vi "Set KH Cluster From UI Array.vi"(8 "error in (no error)":errorcluster, 9 "Number of AI":i32=1, 10 "UI Channels []":T9[](array[typedef]) {"KH"."Channel" items=["A 1"]}, 11 "KH Cluster":T1) -> (0 "error out":errorcluster, 3 "KH Cluster out":T1)   [LabVIEW 2019, in "SMO.Control Experiment UI.lvclass"]
uses:
  SMO.Control Experiment UI.lvclass
  Typedefs/UI Channels--Cluster.ctl
  Typedefs/UI Channels.AI--Cluster.ctl
  Typedefs/UI Channels.Device--Cluster.ctl
  Control Experiment/Typedefs/KH Mode-enum.ctl
  Typedefs/UI Channels.KH--Cluster.ctl
  <userlib>/LevyLab/Krohn Hite 7008/typedefs/Input Configuration-Enum.ctl
  <userlib>/LevyLab/Krohn Hite 7008/typedefs/Gain-Enum.ctl
  <userlib>/LevyLab/Krohn Hite 7008/typedefs/Shunt-Enum.ctl
  Typedefs/UI Channels.AO--Cluster.ctl
  Typedefs/KH Cluster--Cluster.ctl
  <userlib>/LevyLab/Krohn Hite 7008/typedefs/SetAll-Cluster.ctl
  <userlib>/LevyLab/Krohn Hite 7008/typedefs/Channel-Enum.ctl
  <userlib>/LevyLab/Krohn Hite 7008/typedefs/Filter-Enum.ctl
  <userlib>/LevyLab/Krohn Hite 7008/typedefs/Coupling-Enum.ctl
  Control Experiment/Control Experiment.lvclass
  <userlib>/LevyLab/Krohn Hite 7008/Instrument.KH7008.lvclass
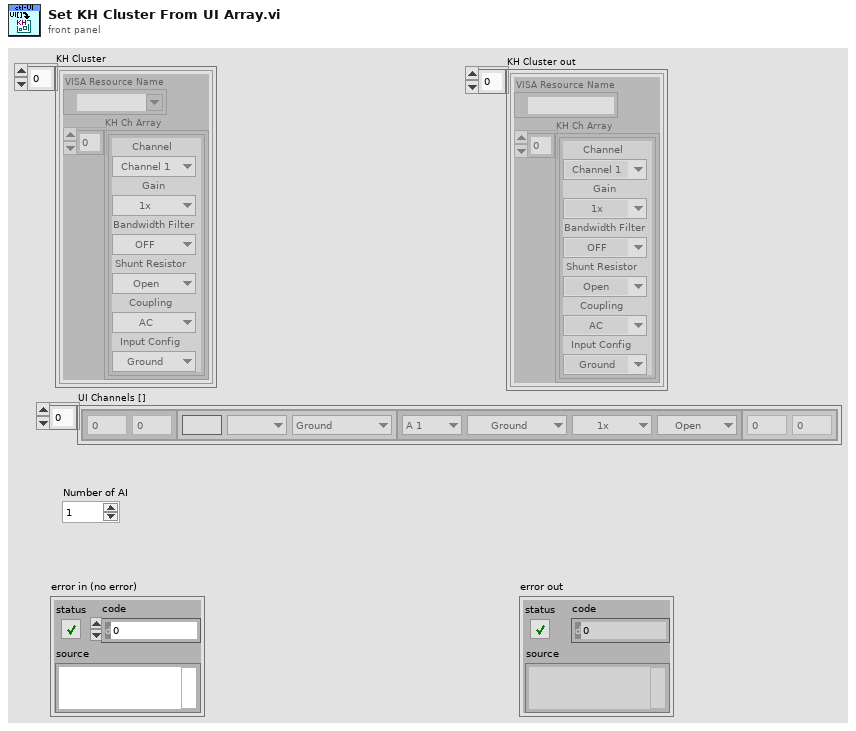
[diagram p1: front panel]
types:
  T1 = typedef "SMO.Control Experiment UI.lvclass/KH Cluster--Cluster.ctl" = cluster{"VISA Resource Name":refnum<visa-resource-name>, "KH Ch Array":T2[]}[]
  T2 = typedef "Instrument.KH7008.lvclass/SetAll-Cluster.ctl" = cluster{"Channel":T3, "Gain":T4, "Bandwidth Filter":T5, "Shunt Resistor":T6, "Coupling":T7, "Input Config":T8}
  T3 = typedef "Instrument.KH7008.lvclass/Channel-Enum.ctl" = enum16{"Channel 1", "Channel 2", "Channel 3", "Channel 4", "Channel 5", "Channel 6", "Channel 7", "Channel 8"}
  T4 = typedef "Instrument.KH7008.lvclass/Gain-Enum.ctl" = enum16{"1x", "10x", "100x", "1000x"}
  T5 = typedef "Instrument.KH7008.lvclass/Filter-Enum.ctl" = enum16{"OFF", "ON"}
  T6 = typedef "Instrument.KH7008.lvclass/Shunt-Enum.ctl" = enum16{"Open", "50 Ohms", "500 Ohms", "5k Ohms", "50k Ohms", "10M Ohm"}
  T7 = typedef "Instrument.KH7008.lvclass/Coupling-Enum.ctl" = enum16{"AC", "DC"}
  T8 = typedef "Instrument.KH7008.lvclass/Input Configuration-Enum.ctl" = enum16{"Ground", "SE+ (-gnd)", "SE- (+gnd)", "Differential"}
  T9 = typedef "SMO.Control Experiment UI.lvclass/UI Channels--Cluster.ctl" = cluster{"AI":T10, "Device":T11, "KH":T13, "AO":T14}
  T10 = typedef "SMO.Control Experiment UI.lvclass/UI Channels.AI--Cluster.ctl" = cluster{"Channel":u32, "Gain":dbl}
  T11 = typedef "SMO.Control Experiment UI.lvclass/UI Channels.Device--Cluster.ctl" = cluster{"Electrode":string, "Configuration":T12, "Label":u16}
  T12 = typedef "Control Experiment.lvclass/KH Mode-enum.ctl" = enum16{"Ground", "Current", "Voltage (SE)", "Voltage (Diff)", "Gate"}
  T13 = typedef "SMO.Control Experiment UI.lvclass/UI Channels.KH--Cluster.ctl" = cluster{"Channel":u16, "Configuration":T8, "Gain":T4, "Shunt Resistor":T6}
  T14 = typedef "SMO.Control Experiment UI.lvclass/UI Channels.AO--Cluster.ctl" = cluster{"Channel":u32, "Gain":dbl}
  T15 = cluster{"VISA Resource Name":refnum<visa-resource-name>, "KH Ch Array":T2[]}
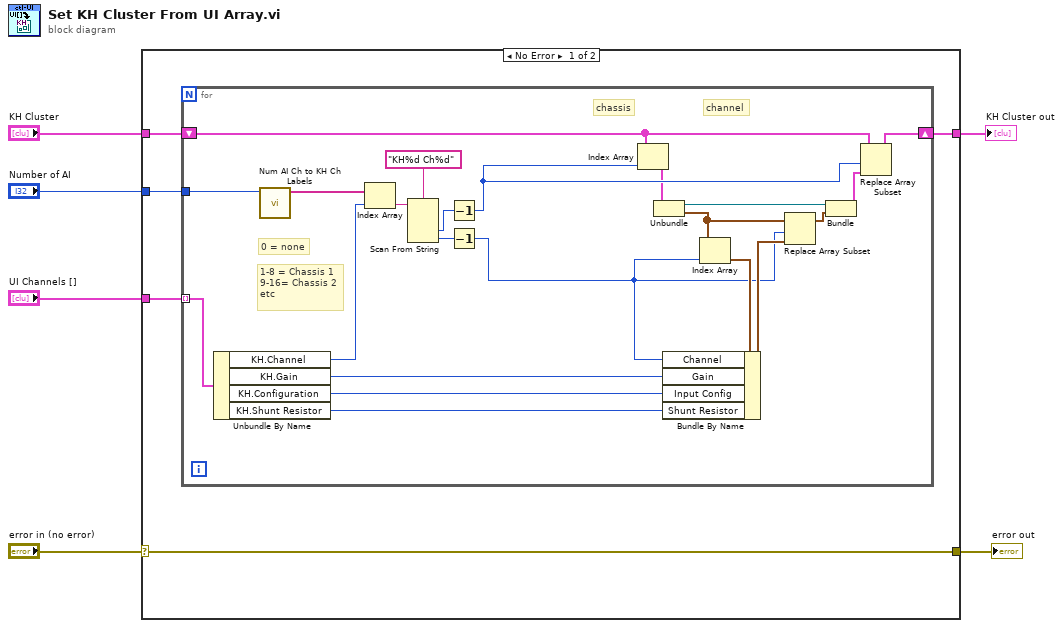
[diagram p0: block diagram]
diagram:
  n1 = case shown="No Error" "error in (no error)" {
    selector: "error in (no error)" -> [w7 w35]
    tunnel: [w11 w34] -> w6
    tunnel: "UI Channels []" -> [w10 _]
    tunnel: "Number of AI" -> [w9 _]
    tunnel: "KH Cluster" -> [w8 w34]
    tunnel: [w7 w35] -> w1
    frame No Error {
      n2 = for {
        tunnel: w10 -> [w20] mode=indexing
        shift-right: [w33] -> w11
        shift-left: w8 -> [w32]
        tunnel: w9 -> [w17]
        # "1-8 = Chassis 1\n9-16= Chassis 2\netc"
        # "0 = none"
        # "channel"
        # "chassis"
        n3 = Unbundle By Name(w20) -> ("KH.Channel"=w19:u16, "KH.Gain"=w21:T4, "KH.Configuration"=w22:T8, "KH.Shunt Resistor"=w23:T6)
        n4 = call "Num AI Ch to KH Ch Labels.vi"("Number of AI"=w17) -> ("KH Ch []"=w18:string[])  [unwired: 9 in, 1 out]
        n5 = Index Array(array=w18, index=w19) -> (element=w29:string)
        n6 = Scan From String(format string="KH%d Ch%d", input string=w29) -> (output 1=w28:i32, output 2=w27:i32)  [unwired: 4 in, 3 out]
        n7 = Decrement(x=w28) -> (x-1=w25:i32)
        n8 = Decrement(x=w27) -> (x-1=w24:i32)
        n9 = Index Array(array=w32, index=w25) -> (element=w15:T15)
        n10 = Unbundle(w15) -> ("VISA Resource Name"=w13:refnum<visa-resource-name>, "KH Ch Array"=w16:T2[])
        n11 = Index Array(array=w16, index=w24) -> (element=w31:T2)
        n12 = Bundle By Name(cluster=w31, "Channel"=w24, "Gain"=w21, "Input Config"=w22, "Shunt Resistor"=w23) -> (w26:T2)
        n13 = Replace Array Subset(array=w16, new element=w26, index=w24) -> (w14:T2[])
        n14 = Bundle("VISA Resource Name"=w13, "KH Ch Array"=w14) -> (w12:T15)  [unwired: 1 in]
        n15 = Replace Array Subset(array=w32, new element=w12, index=w25) -> (w33:T1)
      }
    }
    frame Error {
    }
  }
  "KH Cluster out" <- w6
  "error out" <- w1
